vi "uStringManipulation_removePrefix_Set.vi"(8 "error in (no error)":errorcluster, 10 "prefix":string, 11 "removePrefix in":refnum<class "removePrefix.lvclass">) -> (0 "error out":errorcluster, 3 "removePrefix out":refnum<class "removePrefix.lvclass">)   [LabVIEW 2023, in "uLib.lvlib" / "removePrefix.lvclass"]
doc: "Set a prefix to prepend at the beginning of the string."
uses:
  removePrefix.lvclass
  removePrefix.lvclass/removePrefix.ctl
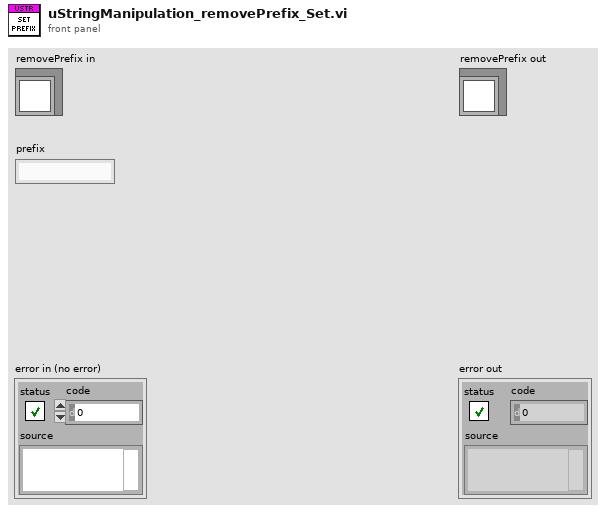
[diagram p1: front panel]
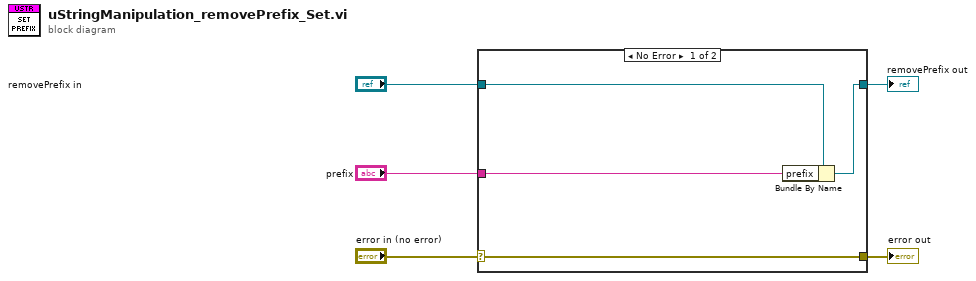
[diagram p0: block diagram]
diagram:
  n1 = case shown="No Error" "error in (no error)" {
    selector: "error in (no error)" -> [w9 w10]
    tunnel: [w9 w10] -> w4
    tunnel: [w7 w11] -> w2
    tunnel: "removePrefix in" -> [w8 w11]
    tunnel: "prefix" -> [w6 _]
    frame No Error {
      n2 = Bundle By Name(cluster=w8, "prefix"=w6) -> (w7:refnum<class "removePrefix.lvclass">)
    }
    frame Error {
    }
  }
  "error out" <- w4
  "removePrefix out" <- w2
